vi "从数据库获取数据通用可配置(子VI).vi"(8 "错误输入（无错误）":errorcluster, 9 "查询参数数组":string[](array[string])=["CODMn", "CODCr", "DO", "铜", "PH", "氨氮", "比电导率", "水温", "COD", "浊度", "总氮", "总磷", "叶绿素a", "藻密度", "水位", "流速", "瞬时流量", "累积流量", "亚硝酸盐", "硫化物", "ORP"], 10 "table输入":string="实时数据", 11 "列队名（唯一）":string) -> (0 "错误输出":errorcluster, 3 "簇数组":cluster{"待发送数据":string[][]}[][](array[cluster]))   [LabVIEW 2016, in "数据传输系统.lvlib"]
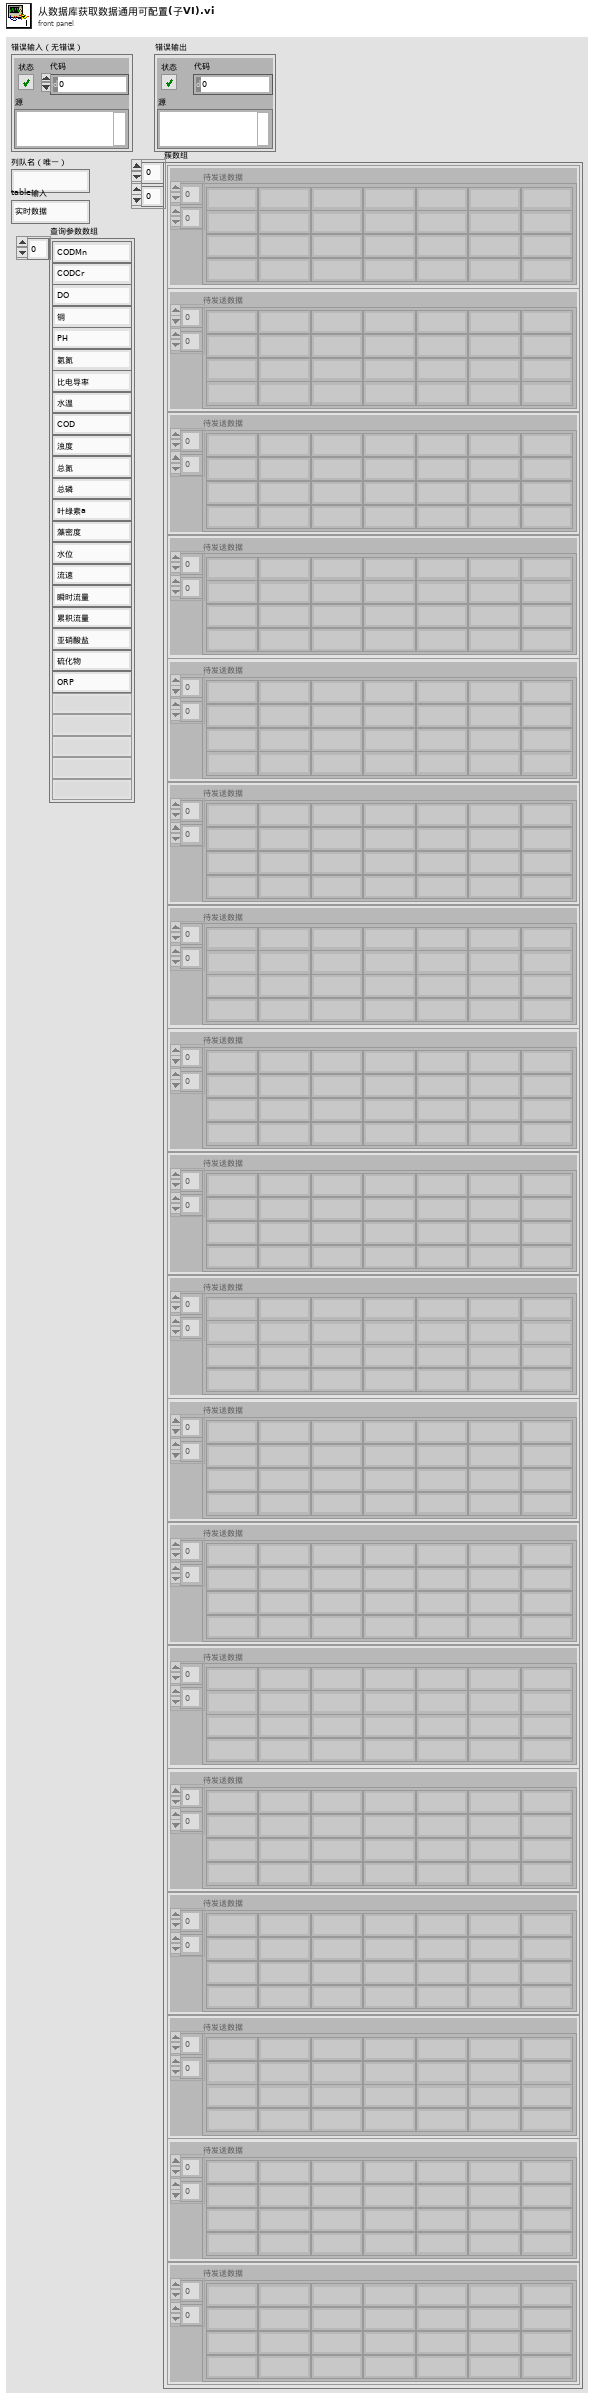
[diagram p1: front panel]
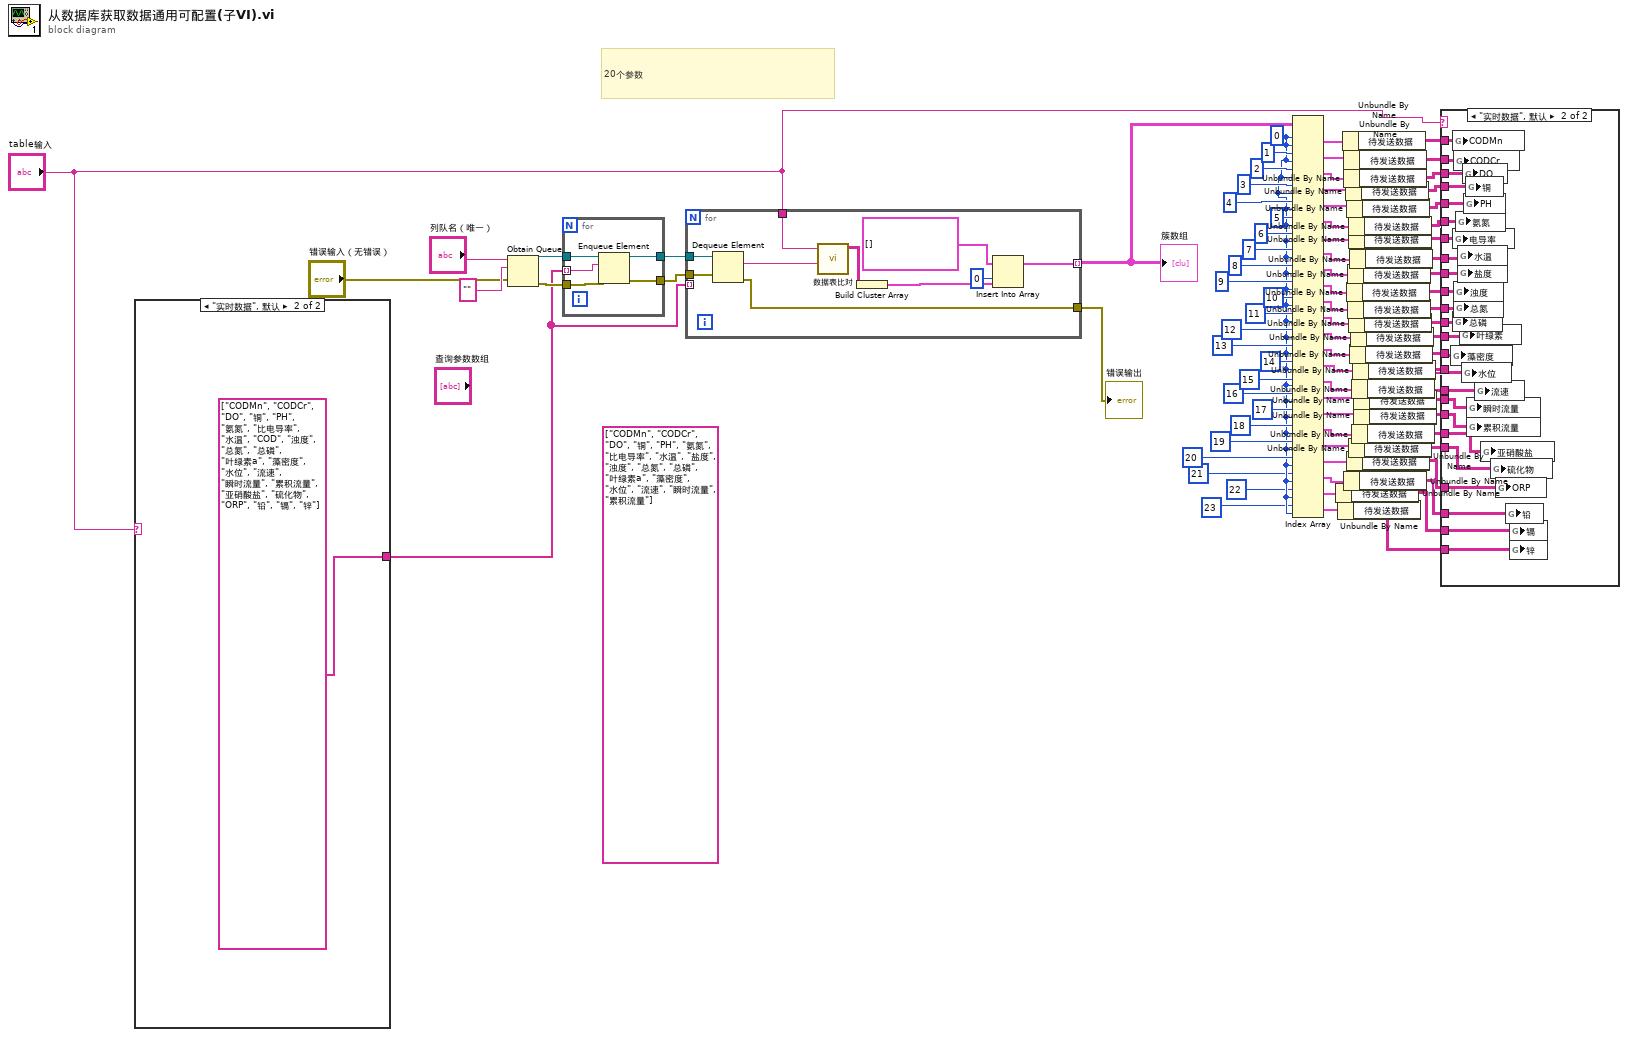
[diagram p0: block diagram]
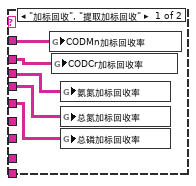
[diagram p2: hidden frame]
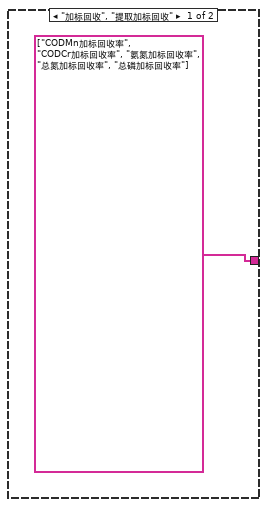
[diagram p3: hidden frame]
diagram:
  (unwired) string[] ["CODMn", "CODCr", "DO", "铜", "PH", "氨氮", "比电导率", "水温", "盐度", "浊度", "总氮", "总磷", "叶绿素a", "藻密度", "水位", "流速", "瞬时流量", "累积流量"] ("查询参数数组")
  w10 = 0 ("索引 (行)")
  # "20个参数"
  n1 = case shown="\"实时数据\", 默认" "table输入" {
    tunnel: [string[] ["CODMn加标回收率", "CODCr加标回收率", "氨氮加标回收率", "总氮加标回收率", "总磷加标回收率"] ("查询参数数组") string[] ["CODMn", "CODCr", "DO", "铜", "PH", "氨氮", "比电导率", "水温", "COD", "浊度", "总氮", "总磷", "叶绿素a", "藻密度", "水位", "流速", "瞬时流量", "累积流量", "亚硝酸盐", "硫化物", "ORP", "铅", "镉", "锌"] ("数组")] -> w33
    frame "加标回收", "提取加标回收" {
    }
    frame "实时数据", Default {
    }
  }
  n2 = Obtain Queue(name (unnamed)="列队名（唯一）", element data type="" ("名称（未命名）"), error in (no error)="错误输入（无错误）") -> (queue out=w81:refnum<queue>, error out=w80:errorcluster)  [unwired: 2 in, 1 out]
  n3 = for {
    tunnel: w33 -> [w88] mode=indexing
    tunnel: w81 -> [w90]
    tunnel: w80 -> [w89]
    tunnel: [w87] -> w79
    tunnel: [w86] -> w78
    n4 = Enqueue Element(queue=w90, element=w88, error in (no error)=w89) -> (queue out=w87:refnum<queue>, error out=w86:errorcluster)  [unwired: 1 in, 1 out]
  }
  n5 = for {
    tunnel: w33 -> [_] mode=indexing
    tunnel: w79 -> [w100]
    tunnel: w78 -> [w99]
    tunnel: [w95] -> w75 mode=indexing
    tunnel: "table输入" -> [w92]
    tunnel: [w91] -> w76
    n6 = Dequeue Element(queue=w100, error in (no error)=w99) -> (element=w98:string, error out=w91:errorcluster)  [unwired: 1 in, 2 out]
    n7 = call "数据表比对.vi"("查询元素输入"=w98, "table输入"=w92) -> ("待发送数据"=w97:string[][])  [unwired: 6 in, 3 out]
    n8 = Build Cluster Array(w97) -> (w96:cluster{"待发送数据":string[][]}[])
    n9 = Insert Into Array(array=cluster{"待发送数据":string[][]}[] [] ("簇数组"), index=0 ("索引"), new element=w96) -> (w95:cluster{"待发送数据":string[][]}[])
  }
  "簇数组" <- w75
  "错误输出" <- w76
  n10 = Index Array(array=w75, index (row) #1=w10, index (col) #1=w10, index (row) #2=1 ("索引 (行)"), index (col) #2=w10, index (row) #3=2 ("索引 (行)"), index (col) #3=w10, index (row) #4=3 ("索引 (行)"), index (col) #4=w10, index (row) #5=4 ("索引 (行)"), index (col) #5=w10, index (row) #6=5 ("索引 (行)"), index (col) #6=w10, index (row) #7=6 ("索引 (行)"), index (col) #7=w10, index (row) #8=7 ("索引 (行)"), index (col) #8=w10, index (row) #9=8 ("索引 (行)"), index (col) #9=w10, index (row) #10=9 ("索引 (行)"), index (col) #10=w10, index (row) #11=10 ("索引 (行)"), index (col) #11=w10, index (row) #12=11 ("索引 (行)"), index (col) #12=w10, index (row) #13=12 ("索引 (行)"), index (col) #13=w10, index (row) #14=13 ("索引 (行)"), index (col) #14=w10, index (row) #15=14 ("禁用的索引 (行)"), index (col) #15=w10, index (row) #16=15 ("禁用的索引 (行)"), index (col) #16=w10, index (row) #17=16 ("禁用的索引 (行)"), index (col) #17=w10, index (row) #18=17 ("禁用的索引 (行)"), index (col) #18=w10, index (row) #19=18 ("禁用的索引 (行)"), index (col) #19=w10, index (row) #20=19 ("禁用的索引 (行)"), index (col) #20=w10, index (row) #21=20 ("禁用的索引 (行)"), index (col) #21=w10, index (row) #22=21 ("禁用的索引 (行)"), index (col) #22=w10, index (row) #23=22 ("禁用的索引 (行)"), index (col) #23=w10, index (row) #24=23 ("禁用的索引 (行)"), index (col) #24=w10) -> (element #1=w74:cluster{"待发送数据":string[][]}, element #2=w59:cluster{"待发送数据":string[][]}, element #3=w58:cluster{"待发送数据":string[][]}, element #4=w57:cluster{"待发送数据":string[][]}, element #5=w56:cluster{"待发送数据":string[][]}, element #6=w55:cluster{"待发送数据":string[][]}, element #7=w53:cluster{"待发送数据":string[][]}, element #8=w54:cluster{"待发送数据":string[][]}, element #9=w52:cluster{"待发送数据":string[][]}, element #10=w51:cluster{"待发送数据":string[][]}, element #11=w50:cluster{"待发送数据":string[][]}, element #12=w49:cluster{"待发送数据":string[][]}, element #13=w48:cluster{"待发送数据":string[][]}, element #14=w47:cluster{"待发送数据":string[][]}, element #15=w28:cluster{"待发送数据":string[][]}, element #16=w26:cluster{"待发送数据":string[][]}, element #17=w25:cluster{"待发送数据":string[][]}, element #18=w24:cluster{"待发送数据":string[][]}, element #19=w19:cluster{"待发送数据":string[][]}, element #20=w15:cluster{"待发送数据":string[][]}, element #21=w14:cluster{"待发送数据":string[][]}, element #22=w6:cluster{"待发送数据":string[][]}, element #23=w5:cluster{"待发送数据":string[][]}, element #24=w4:cluster{"待发送数据":string[][]})
  n11 = Unbundle By Name(w5) -> ("待发送数据"=w2:string[][])
  n12 = Unbundle By Name(w4) -> ("待发送数据"=w1:string[][])
  n13 = Unbundle By Name(w74) -> ("待发送数据"=w73:string[][])
  n14 = Unbundle By Name(w59) -> ("待发送数据"=w46:string[][])
  n15 = Unbundle By Name(w58) -> ("待发送数据"=w45:string[][])
  n16 = Unbundle By Name(w6) -> ("待发送数据"=w3:string[][])
  n17 = Unbundle By Name(w57) -> ("待发送数据"=w44:string[][])
  n18 = Unbundle By Name(w56) -> ("待发送数据"=w43:string[][])
  n19 = Unbundle By Name(w51) -> ("待发送数据"=w38:string[][])
  n20 = Unbundle By Name(w14) -> ("待发送数据"=w11:string[][])
  n21 = Unbundle By Name(w52) -> ("待发送数据"=w39:string[][])
  n22 = Unbundle By Name(w50) -> ("待发送数据"=w37:string[][])
  n23 = Unbundle By Name(w55) -> ("待发送数据"=w42:string[][])
  n24 = Unbundle By Name(w53) -> ("待发送数据"=w41:string[][])
  n25 = Unbundle By Name(w49) -> ("待发送数据"=w36:string[][])
  n26 = Unbundle By Name(w15) -> ("待发送数据"=w12:string[][])
  n27 = Unbundle By Name(w54) -> ("待发送数据"=w40:string[][])
  n28 = Unbundle By Name(w47) -> ("待发送数据"=w35:string[][])
  n29 = Unbundle By Name(w48) -> ("待发送数据"=w34:string[][])
  n30 = Unbundle By Name(w26) -> ("待发送数据"=w23:string[][])
  n31 = Unbundle By Name(w19) -> ("待发送数据"=w13:string[][])
  n32 = Unbundle By Name(w28) -> ("待发送数据"=w27:string[][])
  n33 = Unbundle By Name(w25) -> ("待发送数据"=w22:string[][])
  n34 = Unbundle By Name(w24) -> ("待发送数据"=w21:string[][])
  n35 = case shown="\"实时数据\", 默认" "table输入" {
    tunnel: w73 -> [w105 w129]
    tunnel: w46 -> [w104 w128]
    tunnel: w45 -> [w103 w127]
    tunnel: w44 -> [w102 w126]
    tunnel: w43 -> [w101 w125]
    tunnel: w42 -> [_ w124]
    tunnel: w41 -> [_ w123]
    tunnel: w40 -> [_ w122]
    tunnel: w39 -> [_ w121]
    tunnel: w38 -> [_ w120]
    tunnel: w37 -> [_ w119]
    tunnel: w36 -> [_ w118]
    tunnel: w35 -> [_ w117]
    tunnel: w34 -> [_ w116]
    tunnel: w27 -> [_ w115]
    tunnel: w23 -> [_ w114]
    tunnel: w22 -> [_ w113]
    tunnel: w21 -> [_ w112]
    tunnel: w13 -> [_ w111]
    tunnel: w12 -> [_ w110]
    tunnel: w11 -> [_ w109]
    tunnel: w3 -> [_ w108]
    tunnel: w2 -> [_ w107]
    tunnel: w1 -> [_ w106]
    frame "加标回收", "提取加标回收" {
      n36 = global write "全局 所有参数.vi" "CODMn加标回收率"(w105) -> ()
      n37 = global write "全局 所有参数.vi" "CODCr加标回收率"(w104) -> ()
      n38 = global write "全局 所有参数.vi" "氨氮加标回收率"(w103) -> ()
      n39 = global write "全局 所有参数.vi" "总氮加标回收率"(w102) -> ()
      n40 = global write "全局 所有参数.vi" "总磷加标回收率"(w101) -> ()
    }
    frame "实时数据", Default {
      n41 = global write "全局 所有参数.vi" "藻密度"(w117) -> ()
      n42 = global write "全局 所有参数.vi" "CODMn"(w129) -> ()
      n43 = global write "全局 所有参数.vi" "电导率"(w123) -> ()
      n44 = global write "全局 所有参数.vi" "总磷"(w118) -> ()
      n45 = global write "全局 所有参数.vi" "CODCr"(w128) -> ()
      n46 = global write "全局 所有参数.vi" "浊度"(w120) -> ()
      n47 = global write "全局 所有参数.vi" "总氮"(w119) -> ()
      n48 = global write "全局 所有参数.vi" "氨氮"(w124) -> ()
      n49 = global write "全局 所有参数.vi" "水温"(w122) -> ()
      n50 = global write "全局 所有参数.vi" "盐度"(w121) -> ()
      n51 = global write "全局 所有参数.vi" "叶绿素"(w116) -> ()
      n52 = global write "全局 所有参数.vi" "水位"(w115) -> ()
      n53 = global write "全局 所有参数.vi" "DO"(w127) -> ()
      n54 = global write "全局 所有参数.vi" "PH"(w125) -> ()
      n55 = global write "全局 所有参数.vi" "铜"(w126) -> ()
      n56 = global write "全局 所有参数.vi" "瞬时流量"(w113) -> ()
      n57 = global write "全局 所有参数.vi" "累积流量"(w112) -> ()
      n58 = global write "全局 所有参数.vi" "流速"(w114) -> ()
      n59 = global write "全局 所有参数.vi" "亚硝酸盐"(w111) -> ()
      n60 = global write "全局 所有参数.vi" "硫化物"(w110) -> ()
      n61 = global write "全局 所有参数.vi" "ORP"(w109) -> ()
      n62 = global write "全局 所有参数.vi" "铅"(w108) -> ()
      n63 = global write "全局 所有参数.vi" "镉"(w107) -> ()
      n64 = global write "全局 所有参数.vi" "锌"(w106) -> ()
    }
  }
